vi "LC_BESS_Act_Ctrl.vi"   [LabVIEW 2016]
doc: "-----------------------------------------------------------------------------------------------------------------------\nCopyright <2019> <The University of Tennessee at Knoxville and the University of Tennessee Research Foundation>\nThis software is released under BSD-3\nhttps://opensource.org/licenses/BSD-3-Clause \nAdditional license options available at https://utrf.tennessee.edu/industry/sample-agreements/\n-----------------------------------------------------------------------------------------------------------------------\n\n\nActive power support for BESS local controller"
uses:
  <vilib>/ptbypt/NI_PtbyPt.lvlib
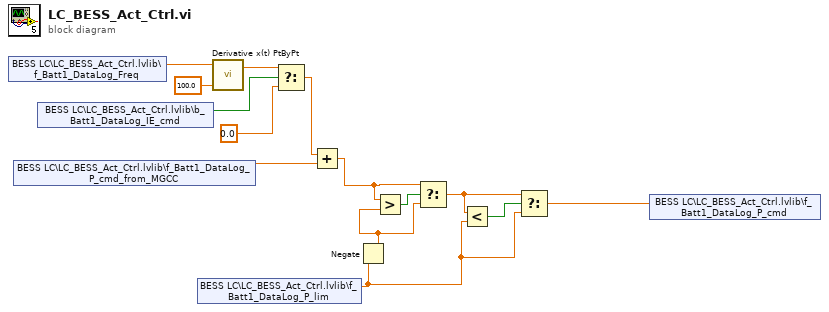
[diagram p0: block diagram]
diagram:
  n1 = shared-variable "BESS LC\\LC_BESS_Act_Ctrl.lvlib\\f_Batt1_DataLog_Freq"() -> (w4:dbl)  [unwired: 1 in, 1 out]
  n2 = shared-variable "BESS LC\\LC_BESS_Act_Ctrl.lvlib\\f_Batt1_DataLog_P_cmd_from_MGCC"() -> (w8:dbl)  [unwired: 1 in, 1 out]
  n3 = shared-variable "BESS LC\\LC_BESS_Act_Ctrl.lvlib\\b_Batt1_DataLog_IE_cmd"() -> (w7:bool)  [unwired: 1 in, 1 out]
  n4 = shared-variable "BESS LC\\LC_BESS_Act_Ctrl.lvlib\\f_Batt1_DataLog_P_lim"() -> (w11:dbl)  [unwired: 1 in, 1 out]
  n5 = call <vilib>:"Derivative x(t) PtByPt.vi"("dt"=100.0, "x"=w4) -> ("dx/dt"=w2:dbl)  [unwired: 2 in, 1 out]
  n6 = Select(t=w2, s=w7, f=0.0) -> (s? t:f=w5:dbl)
  n7 = Add(x=w5, y=w8) -> (x+y=w9:dbl)
  n8 = Negate(x=w11) -> (-x=w13:dbl)
  n9 = Greater?(x=w9, y=w13) -> (0:w14:bool)
  n10 = Select(t=w9, s=w14, f=w13) -> (s? t:f=w12:dbl)
  n11 = Less?(x=w12, y=w11) -> (x < y?=w10:bool)
  n12 = Select(t=w12, s=w10, f=w11) -> (s? t:f=w1:dbl)
  n13 = shared-variable "BESS LC\\LC_BESS_Act_Ctrl.lvlib\\f_Batt1_DataLog_P_cmd"(w1) -> ()  [unwired: 1 in, 1 out]
